vi "Item.vi"(8 "error in (no error)":errorcluster, 10 "Index":i32, 11 "StringList in":refnum<class "StringList.lvclass">) -> (0 "error out":errorcluster, 1 "String":string, 3 "StringList out":refnum<class "StringList.lvclass">)   [LabVIEW 2013, in "LapDog.Collections.v_.Lists.lvlib" / "StringList.lvclass"]
uses:
  StringList.lvclass
  ObjectList/ObjectList.lvclass
  LapDog.Collections.Common/String/String.lvclass
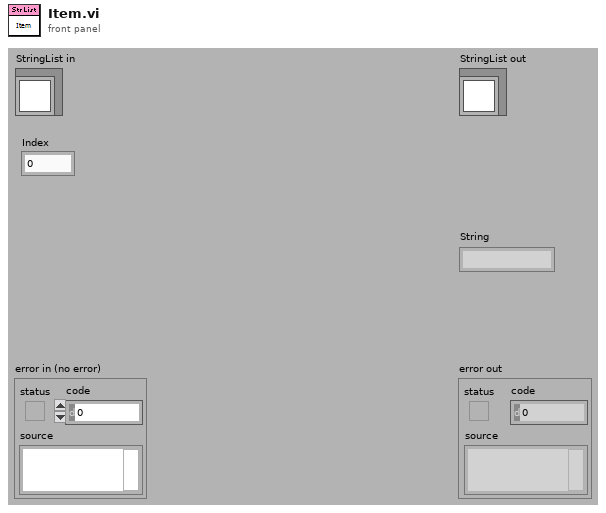
[diagram p1: front panel]
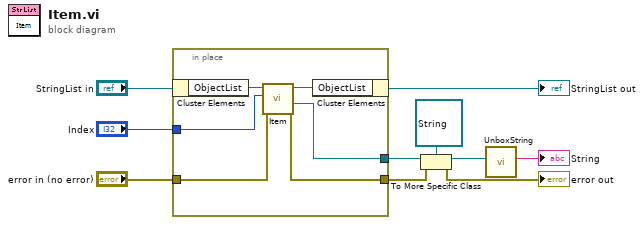
[diagram p0: block diagram]
diagram:
  n1 = in-place {
    in-place-border: "error in (no error)" -> [w14]
    in-place-border: [w13] -> w5
    in-place-border: "Index" -> [w12]
    in-place-border: [w11] -> w4
    n2 = in-place-cluster #1("StringList in") -> ("ObjectList"=w16:refnum<class "ObjectList.lvclass">)
    n3 = call-dynamic "Item.vi"("error in (no error)"=w14, "Index"=w12, "List in"=w16) -> ("error out"=w13:errorcluster, "Item"=w11:refnum<class>, "List out"=w15:refnum<class "ObjectList.lvclass">)  [unwired: 6 in]
    n4 = in-place-cluster #1("ObjectList"=w15) -> (→"StringList out":refnum<class "StringList.lvclass">)
  }
  n5 = To More Specific Class(target class=refnum<class "String.lvclass"> refnum ("LapDog.Collections.v0.Lists.Interfaces.lvlib:String.lvclass"), reference=w4, error in=w5) -> (specific class reference=w2:refnum<class "String.lvclass">, error out=→"error out":errorcluster)
  n6 = call "UnboxString.vi"("String in"=w2) -> ("String"=→"String":string)  [unwired: 10 in]
